vi "SSH Execute Command Wrapper.vi"(8 "Error In":errorcluster, 10 "Command":string, 11 "Install LV Data in":T1) -> (0 "Error Out":errorcluster, 2 "Std Out":string, 3 "Install LV Data out":T1)   [LabVIEW 2020, in "LMH-LINX.lvlib"]
uses:
  LMH-LINX.lvlib
  Target Management/Install LV Data.ctl
  Target Management/Target Info.ctl
  Target Management/NIC Info.ctl
  Target Management/NIC Mode.ctl
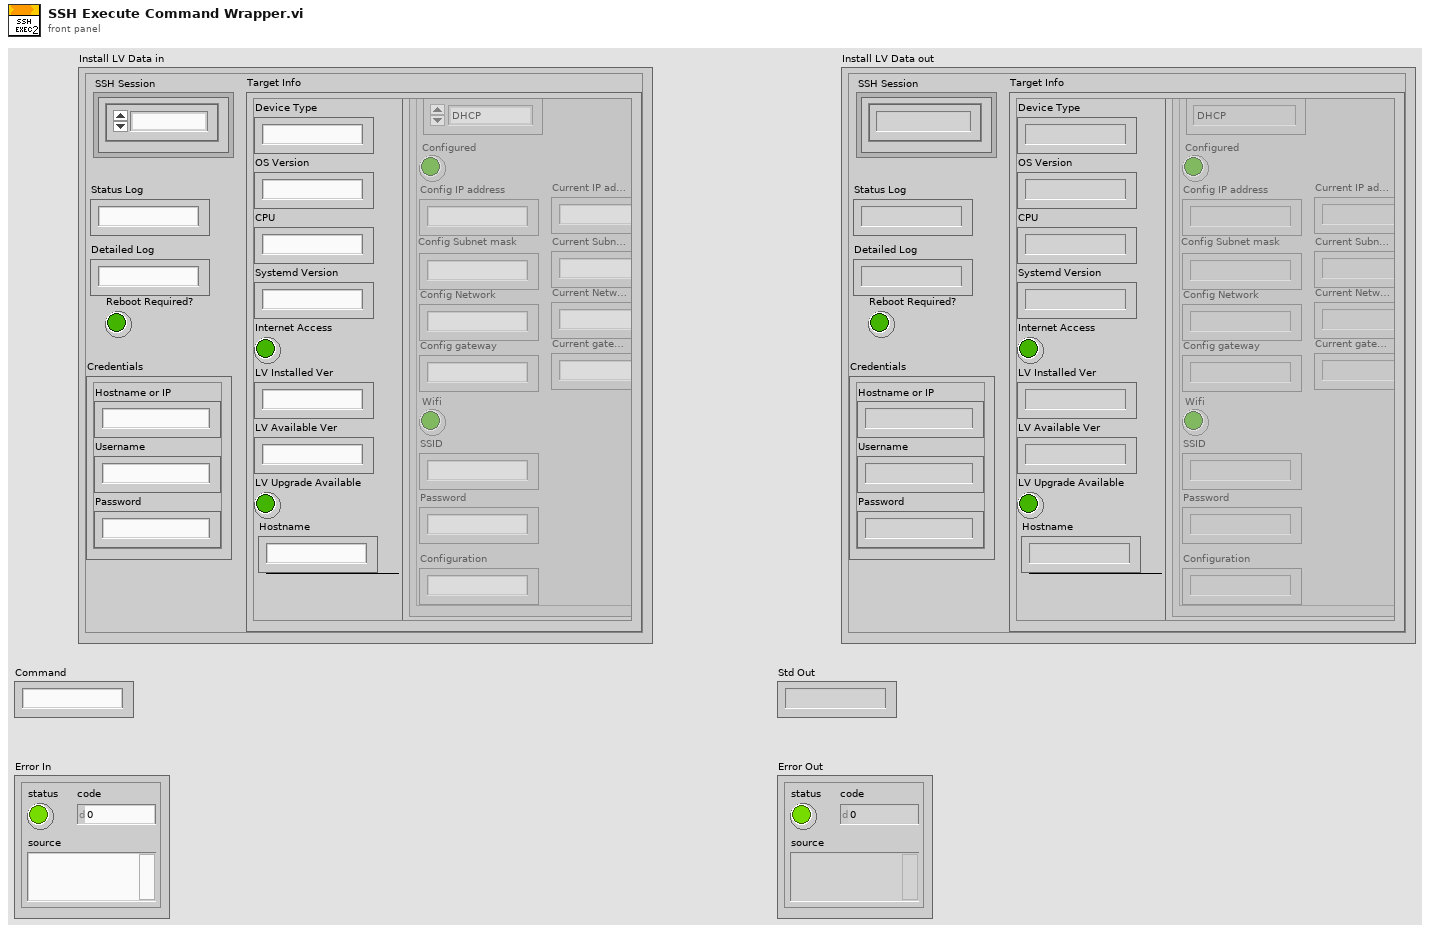
[diagram p1: front panel]
types:
  T1 = typedef "LMH-LINX.lvlib/Install LV Data.ctl" = cluster{"SSH Session":refnum<k1>, "Status Log":string, "Detailed Log":string, "Credentials":cluster{"Hostname or IP":string, "Username":string, "Password":string}, "Target Info":T2, "Reboot Required?":bool}
  T2 = typedef "LMH-LINX.lvlib/Target Info.ctl" = cluster{"OS Version":string, "CPU":string, "Systemd Version":string, "Internet Access":bool, "Device Type":string, "LV Installed Ver":string, "LV Available Ver":string, "LV Upgrade Available":bool, "Hostname":string, "NIC Info":T3[]}
  T3 = typedef "LMH-LINX.lvlib/NIC Info.ctl" = cluster{"Name":string, "NIC Mode":T4, "Configured":bool, "Config IP address":string, "Config Subnet mask":string, "Config Network":string, "Config gateway":string, "Wifi":bool, "SSID":string, "Password":string, "Configuration":string, "Current IP address":string, "Current Subnet mask":string, "Current gateway":string, "Current Network":string}
  T4 = typedef "LMH-LINX.lvlib/NIC Mode.ctl" = enum16{"DHCP", "Static", "Loopback"}
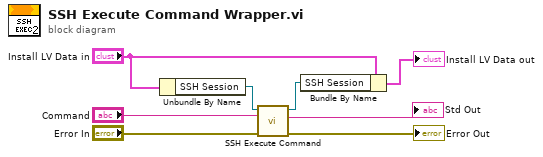
[diagram p0: block diagram]
diagram:
  n1 = Unbundle By Name("Install LV Data in") -> ("SSH Session"=w1:refnum<k1>)
  n2 = call "SSH Execute Command.vi"("Error In"="Error In", "Command"="Command", "SSH Session"=w1) -> ("Error Out"=→"Error Out":errorcluster, "Std Out"=→"Std Out":string, "SSH Session"=w2:refnum<k1>)  [unwired: 6 in]
  n3 = Bundle By Name(cluster="Install LV Data in", "SSH Session"=w2) -> (→"Install LV Data out":T1)
